vi "LEDC Control Loop 2936 Main SA.vi"(0 "LEDAD Port":refnum<visa-resource-name>="COM7", 1 "Enable":u8, 2 "Channel":enum16{"Chn1", "Chn2"}(ring), 5 "Light Meter Port":refnum<visa-resource-name>="COM4", 7 "Illum Desired":dbl, 9 "Error Margin":dbl=2.0, 11 "error in (no error)":errorcluster, 12 "Illum Cal Factor":dbl=3.62982 format="%#.6f", 13 "Stop":bool) -> (3 "In Progress":bool, 4 "LEDAD Port out":refnum<visa-resource-name>, 6 "Light Meter Port out":refnum<visa-resource-name>, 8 "Illum Meas":dbl format="%#_4g", 10 "Inten Desired":dbl, 14 "Done":bool, 15 "error out":errorcluster)   [LabVIEW 2010]
panel:
  out "Flag2":bool
  out "Flag1":bool
  out "Slope":dbl format="%#_4g"
  in  "Illum 10":dbl format="%#_4g"
  in  "Illum 90":dbl format="%#_4g"
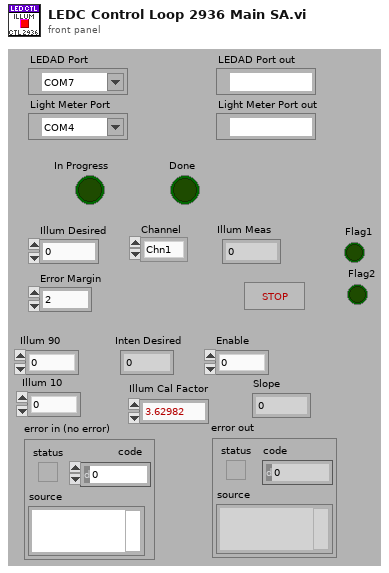
[diagram p1: front panel]
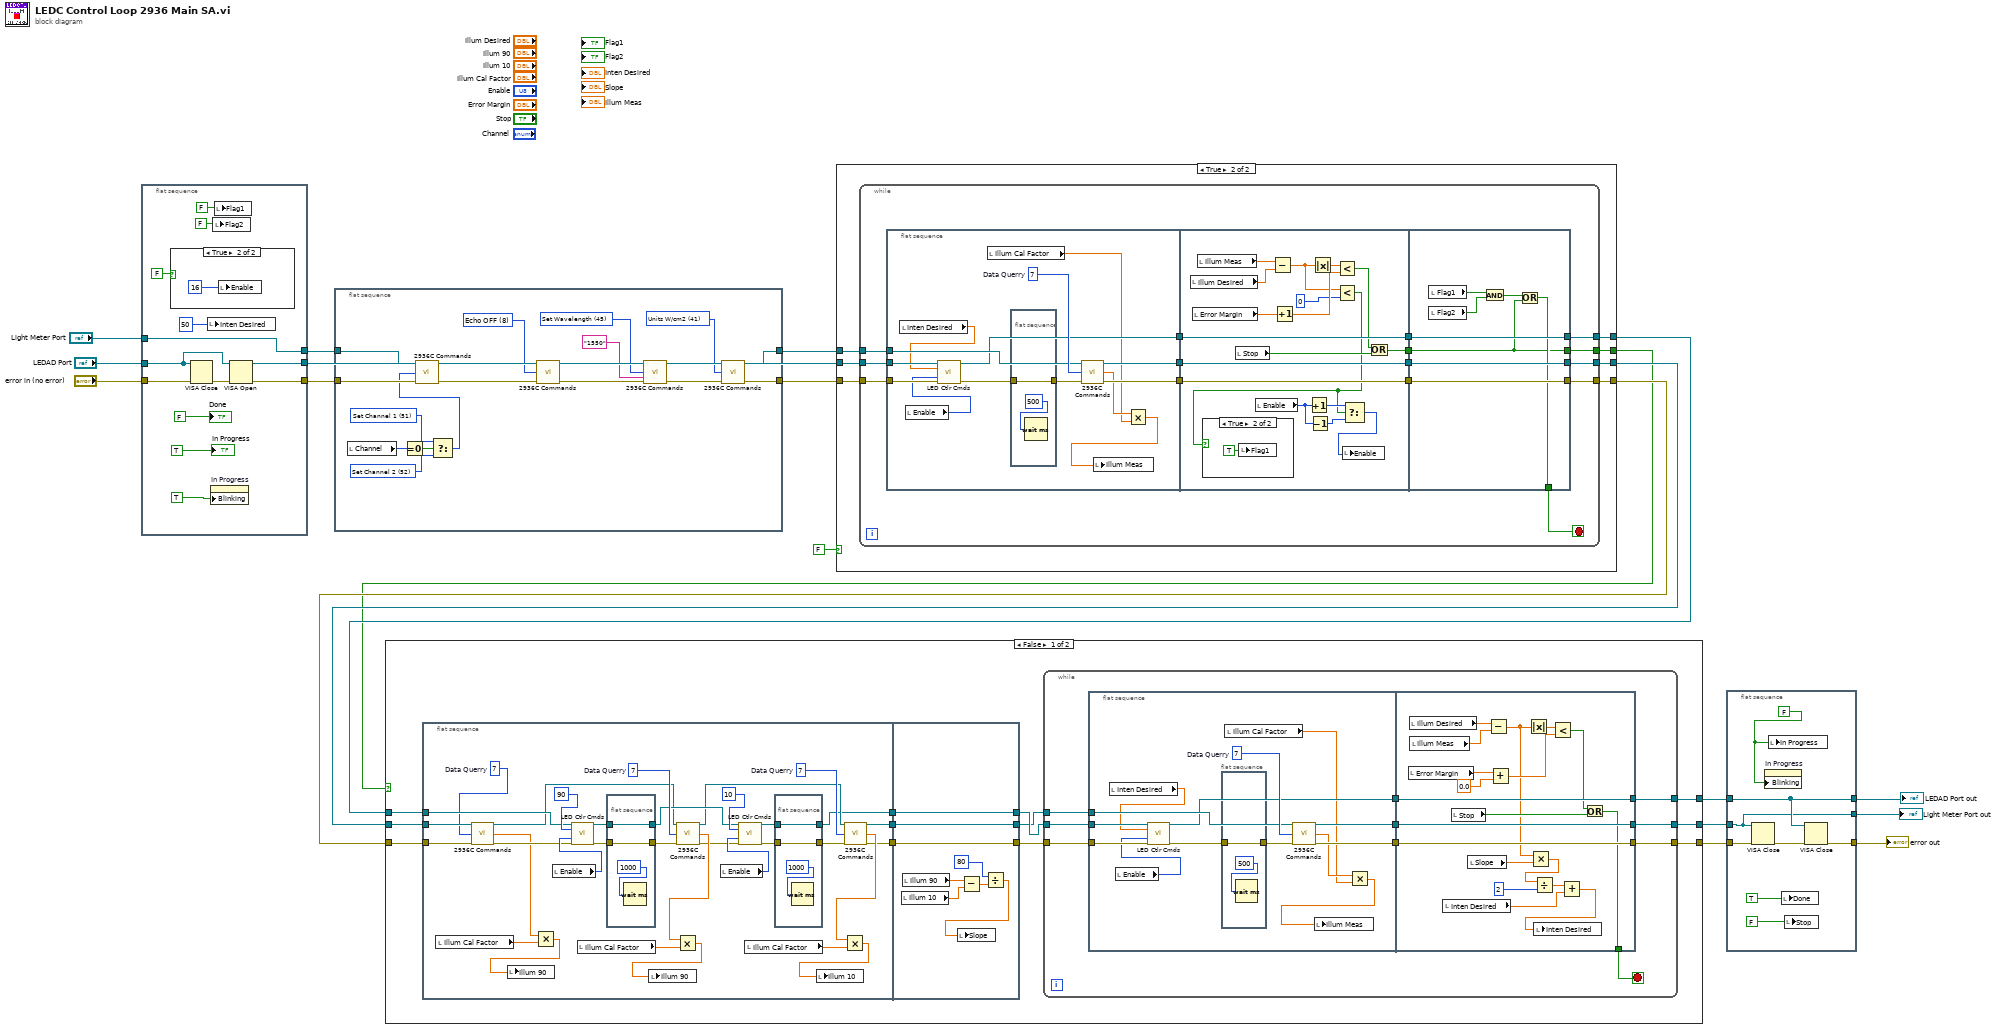
[diagram p0: block diagram]
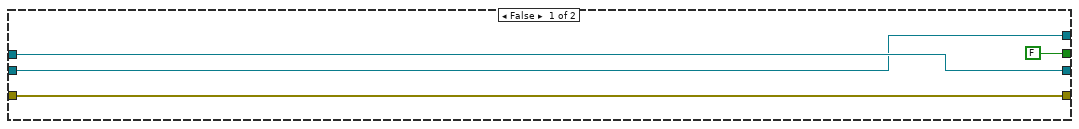
[diagram p2: hidden frame]
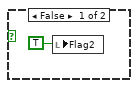
[diagram p3: hidden frame]
diagram:
  n1 = flat-sequence {
    tunnel: "LEDAD Port" -> [w25]
    tunnel: [w27] -> w5
    tunnel: "error in (no error)" -> [w28]
    tunnel: [w26] -> w3
    tunnel: "Light Meter Port" -> [w24]
    tunnel: [w24] -> w2
    frame #0 {
      n2 = case shown="True" FALSE {
        frame False {
        }
        frame True {
          n3 = local write "Enable"(16) -> ()
        }
      }
      n4 = VISA Close(VISA resource name=w25, error in (no error)=w28) -> (error out=w29:errorcluster)
      n5 = local write "Inten Desired"(50) -> ()
      n6 = property on="In Progress" class="Bool (strict)"("Blinking"=TRUE) -> ()  [unwired: 2 in, 2 out]
      n7 = local write "Flag2"(FALSE) -> ()
      n8 = local write "Flag1"(FALSE) -> ()
      n9 = VISA Open(error in (no error)=w29, VISA resource name=w25) -> (VISA resource name=w26:refnum<visa-resource-name>, error out=w27:errorcluster)  [unwired: 3 in]
      "Done" <- FALSE
      "In Progress" <- TRUE
    }
  }
  n10 = flat-sequence {
    tunnel: w5 -> [w52]
    tunnel: [w42] -> w4
    tunnel: w2 -> [w46]
    tunnel: [w45] -> w1
    frame #0 {
      w34 = u16 8 items=["Attenuator OFF", "Attenuator ON", "Attenuator Query", "Beep OFF", "Beep ON", "Beep Query", "Clear Status Reg", "Get Power (nW)", "Echo OFF", "Echo ON", "Echo Query", "No Filter", "Analog Filter", "Digital FIlter", "Filter Query", "Hold", "Go", "Go Query", "Backlight OFF", "Backlight Medium", "Backlight High", "Backlight Query", "Set Dsplay Screen 0", "Set Display Screen 1", "Display Screen Query", "Mode DC Continuous", "Mode DC Single", "Mode Integrate", "Identification", "Auto Range", "Auto Range Query", "Signal Range 0", "Signal Range 1", "Signal Range 2", "Signal Range 3", "Signal Range 4", "Signal Range 5", "Signal Range 6", "Signal Range Query", "Store Reference", "Units W", "Units W/cm2", "Units dBm", "Units Joules", "Units Query", "Set Wavelength", "Wavelength Querry", "Mode Pesk-to-Peak Cont.", "Mode Peak-to-Peak Sing.", "Mode Query", "Channel Querry", "Set Channel 1", "Set Channel 2"] ("Command")
      w39 = u16 41 items=["Attenuator OFF", "Attenuator ON", "Attenuator Query", "Beep OFF", "Beep ON", "Beep Query", "Clear Status Reg", "Get Power (nW)", "Echo OFF", "Echo ON", "Echo Query", "No Filter", "Analog Filter", "Digital FIlter", "Filter Query", "Hold", "Go", "Go Query", "Backlight OFF", "Backlight Medium", "Backlight High", "Backlight Query", "Set Dsplay Screen 0", "Set Display Screen 1", "Display Screen Query", "Mode DC Continuous", "Mode DC Single", "Mode Integrate", "Identification", "Auto Range", "Auto Range Query", "Signal Range 0", "Signal Range 1", "Signal Range 2", "Signal Range 3", "Signal Range 4", "Signal Range 5", "Signal Range 6", "Signal Range Query", "Store Reference", "Units W", "Units W/cm2", "Units dBm", "Units Joules", "Units Query", "Set Wavelength", "Wavelength Querry", "Mode Pesk-to-Peak Cont.", "Mode Peak-to-Peak Sing.", "Mode Query", "Channel Querry", "Set Channel 1", "Set Channel 2"] ("Command")
      w41 = u16 45 items=["Attenuator OFF", "Attenuator ON", "Attenuator Query", "Beep OFF", "Beep ON", "Beep Query", "Clear Status Reg", "Get Power (nW)", "Echo OFF", "Echo ON", "Echo Query", "No Filter", "Analog Filter", "Digital FIlter", "Filter Query", "Hold", "Go", "Go Query", "Backlight OFF", "Backlight Medium", "Backlight High", "Backlight Query", "Set Dsplay Screen 0", "Set Display Screen 1", "Display Screen Query", "Mode DC Continuous", "Mode DC Single", "Mode Integrate", "Identification", "Auto Range", "Auto Range Query", "Signal Range 0", "Signal Range 1", "Signal Range 2", "Signal Range 3", "Signal Range 4", "Signal Range 5", "Signal Range 6", "Signal Range Query", "Store Reference", "Units W", "Units W/cm2", "Units dBm", "Units Joules", "Units Query", "Set Wavelength", "Wavelength Querry", "Mode Pesk-to-Peak Cont.", "Mode Peak-to-Peak Sing.", "Mode Query", "Channel Querry", "Set Channel 1", "Set Channel 2"] ("Command")
      w51 = u16 52 items=["Attenuator OFF", "Attenuator ON", "Attenuator Query", "Beep OFF", "Beep ON", "Beep Query", "Clear Status Reg", "Get Power (nW)", "Echo OFF", "Echo ON", "Echo Query", "No Filter", "Analog Filter", "Digital FIlter", "Filter Query", "Hold", "Go", "Go Query", "Backlight OFF", "Backlight Medium", "Backlight High", "Backlight Query", "Set Dsplay Screen 0", "Set Display Screen 1", "Display Screen Query", "Mode DC Continuous", "Mode DC Single", "Mode Integrate", "Identification", "Auto Range", "Auto Range Query", "Signal Range 0", "Signal Range 1", "Signal Range 2", "Signal Range 3", "Signal Range 4", "Signal Range 5", "Signal Range 6", "Signal Range Query", "Store Reference", "Units W", "Units W/cm2", "Units dBm", "Units Joules", "Units Query", "Set Wavelength", "Wavelength Querry", "Mode Pesk-to-Peak Cont.", "Mode Peak-to-Peak Sing.", "Mode Query", "Channel Querry", "Set Channel 1", "Set Channel 2"] ("Command")
      w50 = u16 51 items=["Attenuator OFF", "Attenuator ON", "Attenuator Query", "Beep OFF", "Beep ON", "Beep Query", "Clear Status Reg", "Get Power (nW)", "Echo OFF", "Echo ON", "Echo Query", "No Filter", "Analog Filter", "Digital FIlter", "Filter Query", "Hold", "Go", "Go Query", "Backlight OFF", "Backlight Medium", "Backlight High", "Backlight Query", "Set Dsplay Screen 0", "Set Display Screen 1", "Display Screen Query", "Mode DC Continuous", "Mode DC Single", "Mode Integrate", "Identification", "Auto Range", "Auto Range Query", "Signal Range 0", "Signal Range 1", "Signal Range 2", "Signal Range 3", "Signal Range 4", "Signal Range 5", "Signal Range 6", "Signal Range Query", "Store Reference", "Units W", "Units W/cm2", "Units dBm", "Units Joules", "Units Query", "Set Wavelength", "Wavelength Querry", "Mode Pesk-to-Peak Cont.", "Mode Peak-to-Peak Sing.", "Mode Query", "Channel Querry", "Set Channel 1", "Set Channel 2"] ("Command")
      n11 = local read "Channel"() -> (w48:enum16{"Chn1", "Chn2"})
      n12 = Equal To 0?(x=w48) -> (x = 0?=w49:bool)
      n13 = Select(t=w50, s=w49, f=w51) -> (s? t:f=w47:u16)
      n14 = call "2936C Commands.vi"("Instrument Resource Name"=w46, "Command"=w47, "error in (no error)"=w52) -> ("VISA resource name out"=w38:refnum<visa-resource-name>, "error out"=w37:errorcluster)  [unwired: 8 in, 3 out]
      n15 = call "2936C Commands.vi"("Instrument Resource Name"=w38, "Command"=w34, "error in (no error)"=w37) -> ("VISA resource name out"=w35:refnum<visa-resource-name>, "error out"=w36:errorcluster)  [unwired: 8 in, 3 out]
      n16 = call "2936C Commands.vi"("Instrument Resource Name"=w35, "Command"=w41, "Wavelength"="1550", "error in (no error)"=w36) -> ("VISA resource name out"=w44:refnum<visa-resource-name>, "error out"=w43:errorcluster)  [unwired: 7 in, 3 out]
      n17 = call "2936C Commands.vi"("Instrument Resource Name"=w44, "Command"=w39, "error in (no error)"=w43) -> ("VISA resource name out"=w45:refnum<visa-resource-name>, "error out"=w42:errorcluster)  [unwired: 8 in, 3 out]
    }
  }
  n18 = case shown="True" FALSE {
    tunnel: w3 -> [w55 w63]
    tunnel: w1 -> [w56 w62]
    tunnel: w4 -> [w54 w61]
    tunnel: [w55 w60] -> w15
    tunnel: [w56 w59] -> w14
    tunnel: [w54 w58] -> w13
    tunnel: [FALSE w57] -> w12
    frame False {
    }
    frame True {
      n19 = while {
        tunnel: w62 -> [w78]
        tunnel: w63 -> [w77]
        tunnel: w61 -> [w76]
        tunnel: [w69] -> w59
        tunnel: [w67] -> w58
        tunnel: [w68] -> w60
        tunnel: [w64] -> w57
        stop <- w65 stop-if-true
        n20 = flat-sequence {
          tunnel: w76 -> [w90]
          tunnel: w77 -> [w91]
          tunnel: w78 -> [w89]
          tunnel: [w88] -> w72
          tunnel: [w86] -> w71
          tunnel: [w87] -> w70
          tunnel: [w111] -> w75
          tunnel: [w110] -> w74
          tunnel: [w109] -> w73
          tunnel: w72 -> [w111]
          tunnel: w71 -> [w110]
          tunnel: w70 -> [w109]
          tunnel: [w96] -> w66
          tunnel: w75 -> [w122]
          tunnel: w74 -> [w121]
          tunnel: w73 -> [w120]
          tunnel: [w122] -> w69
          tunnel: [w121] -> w68
          tunnel: [w120] -> w67
          tunnel: w66 -> [w115]
          tunnel: [w116] -> w65
          tunnel: [w115] -> w64
          frame #0 {
            w92 = 7  # Data Querry
            n21 = local read "Inten Desired"() -> (w83:dbl)
            n22 = local read "Enable"() -> (w82:u8)
            n23 = call "LED Ctlr Cmds.vi"("VISA session"=w91, "Intensity"=w83, "Enable"=w82, "error in (no error)"=w90) -> ("VISA session out"=w86:refnum<visa-resource-name>, "error out"=w85:errorcluster)  [unwired: 7 in, 3 out]
            n24 = local read "Illum Cal Factor"() -> (w79:dbl)
            n25 = flat-sequence {
              tunnel: w85 -> [w94]
              tunnel: [w94] -> w84
              frame #0 {
                n26 = Wait (ms)(milliseconds to wait=500) -> ()  [unwired: 1 out]
              }
            }
            n27 = call "2936C Commands.vi"("Instrument Resource Name"=w89, "Command"=w92, "error in (no error)"=w84) -> ("VISA resource name out"=w88:refnum<visa-resource-name>, "LM Response"=w80:dbl, "error out"=w87:errorcluster)  [unwired: 8 in, 2 out]
            n28 = Multiply(x=w80, y=w79) -> (x*y=w81:dbl)
            n29 = local write "Illum Meas"(w81) -> ()
          }
          frame #1 {
            n30 = local read "Illum Desired"() -> (w106:dbl)
            n31 = local read "Error Margin"() -> (w104:dbl)
            n32 = local read "Illum Meas"() -> (w107:dbl)
            n33 = local read "Stop"() -> (w103:bool)
            n34 = local read "Enable"() -> (w98:u8)
            n35 = Subtract(x=w107, y=w106) -> (x-y=w102:dbl)
            n36 = Increment(x=w104) -> (x+1=w105:dbl)
            n37 = Increment(x=w98) -> (x+1=w99:u8)
            n38 = Decrement(x=w98) -> (x-1=w100:u8)
            n39 = Absolute Value(x=w102) -> (abs(x)=w112:dbl)
            n40 = Less?(x=w112, y=w105) -> (x < y?=w108:bool)
            n41 = Less?(x=w102, y=0) -> (x < y?=w97:bool)
            n42 = case shown="True" w97 {
              frame False {
                n43 = local write "Flag2"(TRUE) -> ()
              }
              frame True {
                n44 = local write "Flag1"(TRUE) -> ()
              }
            }
            n45 = Select(t=w99, s=w97, f=w100) -> (s? t:f=w95:u8)
            n46 = local write "Enable"(w95) -> ()
            n47 = Or(x=w108, y=w103) -> (x .or. y?=w96:bool)
          }
          frame #2 {
            n48 = local read "Flag1"() -> (w119:bool)
            n49 = local read "Flag2"() -> (w118:bool)
            n50 = And(x=w119, y=w118) -> (x .and. y?=w117:bool)
            n51 = Or(x=w117, y=w115) -> (x .or. y?=w116:bool)
          }
        }
      }
    }
  }
  n52 = case shown="False" w12 {
    tunnel: w15 -> [w126 w227]
    tunnel: w14 -> [w132 w228]
    tunnel: w13 -> [w131 w229]
    tunnel: [w127 w229] -> w11
    tunnel: [w129 w228] -> w10
    tunnel: [w128 w227] -> w9
    frame False {
      n53 = flat-sequence {
        tunnel: w132 -> [w142]
        tunnel: w131 -> [w141]
        tunnel: [w148] -> w134
        tunnel: [w147] -> w133
        tunnel: w126 -> [w146]
        tunnel: [w143] -> w125
        tunnel: [w181] -> w123
        tunnel: w134 -> [w181]
        tunnel: [w180] -> w130
        tunnel: w133 -> [w180]
        tunnel: [w176] -> w124
        tunnel: w125 -> [w176]
        frame #0 {
          w138 = 7  # Data Querry
          w155 = 7  # Data Querry
          w162 = 7  # Data Querry
          n54 = local read "Illum Cal Factor"() -> (w137:dbl)
          n55 = call "2936C Commands.vi"("Instrument Resource Name"=w142, "Command"=w138, "error in (no error)"=w141) -> ("VISA resource name out"=w140:refnum<visa-resource-name>, "LM Response"=w135:dbl, "error out"=w139:errorcluster)  [unwired: 8 in, 2 out]
          n56 = Multiply(x=w135, y=w137) -> (x*y=w136:dbl)
          n57 = local write "Illum 90"(w136) -> ()
          n58 = local read "Enable"() -> (w167:u8)
          n59 = call "LED Ctlr Cmds.vi"("VISA session"=w146, "Intensity"=90, "Enable"=w167, "error in (no error)"=w139) -> ("VISA session out"=w164:refnum<visa-resource-name>, "error out"=w165:errorcluster)  [unwired: 7 in, 3 out]
          n60 = local read "Illum Cal Factor"() -> (w159:dbl)
          n61 = flat-sequence {
            tunnel: w165 -> [w173]
            tunnel: [w173] -> w163
            tunnel: [w171] -> w145
            tunnel: w164 -> [w171]
            frame #0 {
              n62 = Wait (ms)(milliseconds to wait=1000) -> ()  [unwired: 1 out]
            }
          }
          n63 = call "2936C Commands.vi"("Instrument Resource Name"=w140, "Command"=w162, "error in (no error)"=w163) -> ("VISA resource name out"=w144:refnum<visa-resource-name>, "LM Response"=w160:dbl, "error out"=w149:errorcluster)  [unwired: 8 in, 2 out]
          n64 = Multiply(x=w160, y=w159) -> (x*y=w161:dbl)
          n65 = local write "Illum 90"(w161) -> ()
          n66 = local read "Enable"() -> (w150:u8)
          n67 = call "LED Ctlr Cmds.vi"("VISA session"=w145, "Intensity"=10, "Enable"=w150, "error in (no error)"=w149) -> ("VISA session out"=w153:refnum<visa-resource-name>, "error out"=w152:errorcluster)  [unwired: 7 in, 3 out]
          n68 = local read "Illum Cal Factor"() -> (w158:dbl)
          n69 = flat-sequence {
            tunnel: w152 -> [w170]
            tunnel: [w170] -> w154
            tunnel: [w168] -> w143
            tunnel: w153 -> [w168]
            frame #0 {
              n70 = Wait (ms)(milliseconds to wait=1000) -> ()  [unwired: 1 out]
            }
          }
          n71 = call "2936C Commands.vi"("Instrument Resource Name"=w144, "Command"=w155, "error in (no error)"=w154) -> ("VISA resource name out"=w148:refnum<visa-resource-name>, "LM Response"=w157:dbl, "error out"=w147:errorcluster)  [unwired: 8 in, 2 out]
          n72 = Multiply(x=w157, y=w158) -> (x*y=w156:dbl)
          n73 = local write "Illum 10"(w156) -> ()
        }
        frame #1 {
          n74 = local read "Illum 10"() -> (w178:dbl)
          n75 = local read "Illum 90"() -> (w179:dbl)
          n76 = Subtract(x=w179, y=w178) -> (x-y=w175:dbl)
          n77 = Divide(x=80, y=w175) -> (x/y=w177:dbl)
          n78 = local write "Slope"(w177) -> ()
        }
      }
      n79 = while {
        tunnel: w123 -> [w191]
        tunnel: w124 -> [w190]
        tunnel: w130 -> [w189]
        tunnel: [w185] -> w129
        tunnel: [w183] -> w127
        tunnel: [w184] -> w128
        stop <- w182 stop-if-true
        n80 = flat-sequence {
          tunnel: w189 -> [w203]
          tunnel: w190 -> [w204]
          tunnel: w191 -> [w202]
          tunnel: [w201] -> w188
          tunnel: [w199] -> w187
          tunnel: [w200] -> w186
          tunnel: w188 -> [w225]
          tunnel: w187 -> [w224]
          tunnel: w186 -> [w223]
          tunnel: [w210] -> w182
          tunnel: [w225] -> w185
          tunnel: [w224] -> w184
          tunnel: [w223] -> w183
          frame #0 {
            w205 = 7  # Data Querry
            n81 = local read "Inten Desired"() -> (w196:dbl)
            n82 = local read "Enable"() -> (w195:u8)
            n83 = call "LED Ctlr Cmds.vi"("VISA session"=w204, "Intensity"=w196, "Enable"=w195, "error in (no error)"=w203) -> ("VISA session out"=w199:refnum<visa-resource-name>, "error out"=w198:errorcluster)  [unwired: 7 in, 3 out]
            n84 = flat-sequence {
              tunnel: w198 -> [w207]
              tunnel: [w207] -> w197
              frame #0 {
                n85 = Wait (ms)(milliseconds to wait=500) -> ()  [unwired: 1 out]
              }
            }
            n86 = local read "Illum Cal Factor"() -> (w192:dbl)
            n87 = call "2936C Commands.vi"("Instrument Resource Name"=w202, "Command"=w205, "error in (no error)"=w197) -> ("VISA resource name out"=w201:refnum<visa-resource-name>, "LM Response"=w193:dbl, "error out"=w200:errorcluster)  [unwired: 8 in, 2 out]
            n88 = Multiply(x=w193, y=w192) -> (x*y=w194:dbl)
            n89 = local write "Illum Meas"(w194) -> ()
          }
          frame #1 {
            n90 = local read "Error Margin"() -> (w209:dbl)
            n91 = local read "Illum Desired"() -> (w221:dbl)
            n92 = local read "Illum Meas"() -> (w220:dbl)
            n93 = local read "Inten Desired"() -> (w212:dbl)
            n94 = local read "Stop"() -> (w218:bool)
            n95 = local read "Slope"() -> (w216:dbl)
            n96 = Subtract(x=w221, y=w220) -> (x-y=w214:dbl)
            n97 = Add(x=w209, y=0.0) -> (x+y=w219:dbl)
            n98 = Absolute Value(x=w214) -> (abs(x)=w226:dbl)
            n99 = Multiply(x=w214, y=w216) -> (x*y=w213:dbl)
            n100 = Divide(x=w213, y=2) -> (x/y=w215:dbl)
            n101 = Less?(x=w226, y=w219) -> (x < y?=w222:bool)
            n102 = Add(x=w215, y=w212) -> (x+y=w211:dbl)
            n103 = local write "Inten Desired"(w211) -> ()
            n104 = Or(x=w222, y=w218) -> (x .or. y?=w210:bool)
          }
        }
      }
    }
    frame True {
    }
  }
  n105 = flat-sequence {
    tunnel: w10 -> [w233]
    tunnel: w11 -> [w235]
    tunnel: [w234] -> w7
    tunnel: w9 -> [w234]
    tunnel: [w233] -> w8
    tunnel: [w231] -> w19
    frame #0 {
      w237 = FALSE
      n106 = VISA Close(VISA resource name=w233, error in (no error)=w235) -> (error out=w232:errorcluster)
      n107 = property on="In Progress" class="Bool (strict)"("Blinking"=w237) -> ()  [unwired: 2 in, 2 out]
      n108 = local write "In Progress"(w237) -> ()
      n109 = local write "Done"(TRUE) -> ()
      n110 = local write "Stop"(FALSE) -> ()
      n111 = VISA Close(VISA resource name=w234, error in (no error)=w232) -> (error out=w231:errorcluster)
    }
  }
  "error out" <- w19
  "Light Meter Port out" <- w8
  "LEDAD Port out" <- w7
